vi "Next Post Processor Name.vi"(7 "Ack Result":refnum<class "Acquired Result.lvclass">, 8 "error in (no error)":errorcluster, 11 "Monitor-Pulse in":refnum<class "Batch Processor.lvclass">) -> (0 "error out":errorcluster, 1 "Complete":bool, 2 "Post processor name":string, 3 "Monitor-Pulse out":refnum<class "Batch Processor.lvclass">, 5 "Ack Result out":refnum<class "Acquired Result.lvclass">)   [LabVIEW 2016, in "Batch Processor.lvclass"]
uses:
  Batch Processor.lvclass
  C:/Github/LabActor/Worker/Worker.lvclass
  C:/Program Files/National Instruments/LabVIEW 2016/vi.lib/ActorFramework/Actor/Actor.lvclass
  C:/Github/LabActor/Template Module/Template Module.lvclass
  NHMFL_Core/Libraries/Instruments/Results/Acquired Result/Acquired Result.lvclass
  Worker/Worker.lvclass/Worker.ctl
  <vilib>/ActorFramework/Actor/Actor.lvclass/Actor.ctl
  <vilib>/ActorFramework/Message Enqueuer/Message Enqueuer.lvclass/Message Enqueuer.ctl
  Process Controller Messages/Update Plots Msg/Update Plots Msg.lvclass/Update Plots Msg.ctl
  NHMFL_Core/Libraries/Instruments/Instrument Driver/Worker State.ctl
  Batch Processor.lvclass/Batch Processor.ctl
  Template Module/Template Module.lvclass/Template Module.ctl
  NHMFL_Core/Libraries/Instruments/Results/File Path Result/File Path Result.lvclass
  C:/Github/NHMFL_Core/Libraries/Instruments/Results/Acquired Result/Acquired Result.lvclass
  Template Module/Read tdms stream.vi
  Template Module/Write State.vi
  Template Module/Read State.vi
  Worker/Read File Path.vi
  <vilib>/ActorFramework/Message Enqueuer/Init from Existing Queue.vi
  <vilib>/ActorFramework/Message Enqueuer/Enqueue.vi
  Process Controller Messages/Update Plots Msg/Update Plots Msg.lvclass
  C:/Program Files/National Instruments/LabVIEW 2016/vi.lib/ActorFramework/Message/Message.lvclass
  <vilib>/ActorFramework/Message Priority Queue/Priority Enqueue.vi
  <vilib>/ActorFramework/Message Enqueuer/Message Enqueuer.lvclass
  Application Controller/Application Controller.lvclass
  <vilib>/ActorFramework/Actor/Actor.lvclass
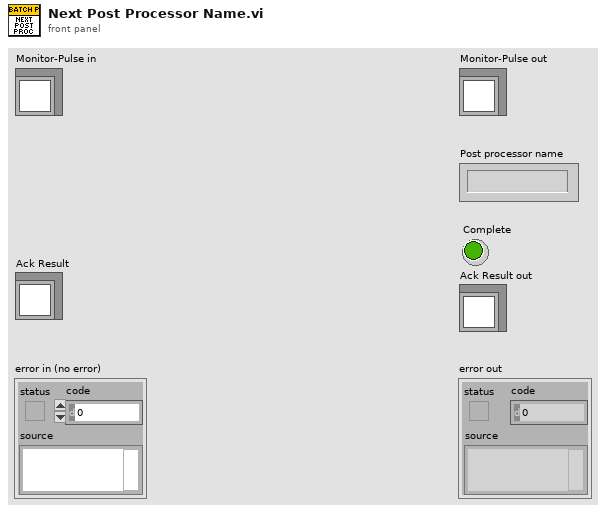
[diagram p1: front panel]
types:
  T1 = typedef "Worker State.ctl" = enum16{"Idle", "Starting", "Working", "Stopping"}
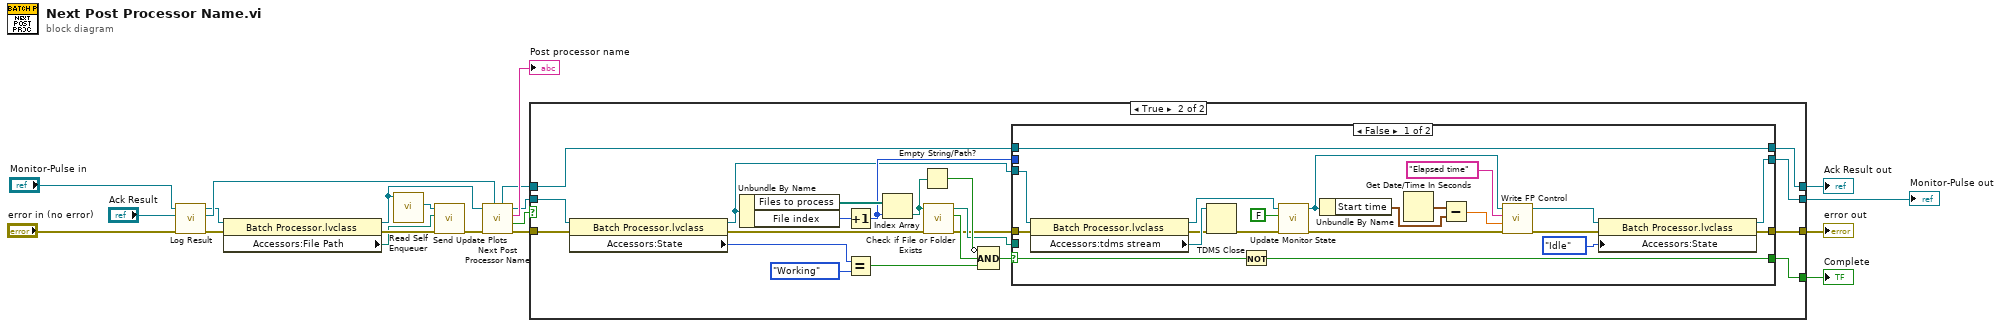
[diagram p0: block diagram]
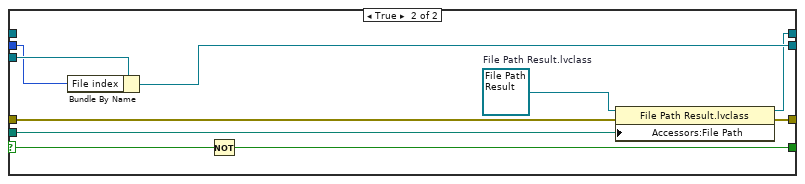
[diagram p3: hidden frame]
diagram:
  n1 = call-dynamic "Log Result.vi"("error in (no error)"="error in (no error)", "Result"="Ack Result", "Process Controller in"="Monitor-Pulse in") -> ("error out"=w9:errorcluster, "Result out"=w3:refnum<class "Acquired Result.lvclass">, "Process Controller out"=w2:refnum<class "Batch Processor.lvclass">)  [unwired: 6 in]
  n2 = property class="Batch Processor.lvclass"(reference=w2, error in=w9) -> (reference out=w1:refnum<class "Batch Processor.lvclass">, error out=w6:errorcluster, "Accessors:File Path"=w4:path)
  n3 = call <vilib>:"Read Self Enqueuer.vi"("Actor"=w1) -> ("Self Enqueuer"=w7:refnum<class "Message Enqueuer.lvclass">)  [unwired: 10 in]
  n4 = call "Send Update Plots.vi"("error in (no error)"=w6, "File Path"=w4, "Message Enqueuer"=w7) -> ("error out"=w5:errorcluster)  [unwired: 7 in, 1 out]
  n5 = call-parent "Next Post Processor Name.vi"("Ack Result"=w3, "error in (no error)"=w5, "Monitor-Pulse in"=w1) -> ("error out"=w19:errorcluster, "Complete"=w17:bool, "Post processor name"=→"Post processor name":string, "Monitor-Pulse out"=w18:refnum<class "Batch Processor.lvclass">, "Ack Result out"=w8:refnum<class "Acquired Result.lvclass">)  [unwired: 4 in]
  n6 = case shown="True" w17 {
    selector: w17 -> [w21 _]
    tunnel: w18 -> [w23 w32]
    tunnel: w19 -> [w24 w30]
    tunnel: [w24 w37] -> w15
    tunnel: [w23 w36] -> w16
    tunnel: w8 -> [w22 w33]
    tunnel: [w22 w35] -> w14
    tunnel: [w21 w34] -> w13
    frame False {
    }
    frame True {
      n7 = property class="Batch Processor.lvclass"(reference=w32, error in=w30) -> (reference out=w31:refnum<class "Batch Processor.lvclass">, error out=w29:errorcluster, "Accessors:State"=w28:T1)
      n8 = Unbundle By Name(w31) -> ("Files to process"=w45:path[], "File index"=w39:i32)
      n9 = Increment(x=w39) -> (x+1=w38:i32)
      n10 = Equal?(x=w28, y=Worker_State."Working") -> (x = y?=w26:bool)
      n11 = Index Array(array=w45, index=w38) -> (element=w44:path)
      n12 = Empty String/Path?(string/path=w44) -> (empty?=w43:bool)
      n13 = call <vilib>:"Check if File or Folder Exists.vi"("error in (no error)"=w29, "path"=w44) -> ("error out"=w40:errorcluster, "file or folder exists?"=w42:bool, "dup path"=w41:path)  [unwired: 7 in]
      n14 = Compound Arithmetic op=AND(invert w43, w42, w26) -> (w25:bool)
      n15 = case shown="False" w25 {
        selector: w25 -> [w58 w69]
        tunnel: w31 -> [w66 w76]
        tunnel: w41 -> [_ w75]
        tunnel: w40 -> [w65 w74]
        tunnel: w38 -> [_ w73]
        tunnel: [w49 w72] -> w37
        tunnel: [w47 w71] -> w36
        tunnel: [w56 w70] -> w35
        tunnel: [w57 w68] -> w34
        tunnel: w33 -> [w56 _]
        frame False {
          n16 = property class="Batch Processor.lvclass"(reference=w66, error in=w65) -> (reference out=w61:refnum<class "Batch Processor.lvclass">, error out=w63:errorcluster, "Accessors:tdms stream"=w64:refnum<k34>)
          n17 = TDMS Close(8:w63, 11:w64) -> (0:w60:errorcluster)  [unwired: 1 out]
          n18 = Not(x=w58) -> (.not. x?=w57:bool)
          n19 = call-dynamic "Update Monitor State.vi"("error in (no error)"=w60, "Monitor Running"=FALSE, "Monitor-Pulse in"=w61) -> ("error out"=w59:errorcluster, "Monitor-Pulse out"=w53:refnum<class "Batch Processor.lvclass">)  [unwired: 7 in]
          n20 = Unbundle By Name(w53) -> ("Start time"=w51:timestamp)
          n21 = Get Date/Time In Seconds() -> (seconds since 1Jan1904=w52:timestamp)
          n22 = Subtract(x=w52, y=w51) -> (x-y=w50:dbl)
          n23 = call-dynamic "Write FP Control.vi"("error in (no error)"=w59, "Control Value"=w50, "Control Name"="Elapsed time", "Measure Object in"=w53) -> ("error out"=w55:errorcluster, "Measure Object out"=w48:refnum<class "Batch Processor.lvclass">)  [unwired: 6 in]
          n24 = property class="Batch Processor.lvclass"(reference=w48, error in=w55, "Accessors:State"=Worker_State."Idle" ("State")) -> (reference out=w47:refnum<class "Batch Processor.lvclass">, error out=w49:errorcluster)
        }
        frame True {
          w67 = refnum<class "File Path Result.lvclass"> refnum  # File Path Result.lvclass
          n25 = Bundle By Name(cluster=w76, "File index"=w73) -> (w71:refnum<class "Batch Processor.lvclass">)
          n26 = Not(x=w69) -> (.not. x?=w68:bool)
          n27 = property class="File Path Result.lvclass"(reference=w67, error in=w74, "Accessors:File Path"=w75) -> (reference out=w70:refnum<class "File Path Result.lvclass">, error out=w72:errorcluster)
        }
      }
    }
  }
  "error out" <- w15
  "Monitor-Pulse out" <- w16
  "Complete" <- w13
  "Ack Result out" <- w14
